vi "M07 Energy Storage.vi"(11 "NXT/EV3":T1) -> (3 "EV3 out":T1)   [LabVIEW 2016]
uses:
  <vilib>/NXT/Subs/LVHSConnector.ctl
  <vilib>/NXT/LegoClasses/BrickReference/BrickReference.lvclass
  <vilib>/NXT/Dual Mode Library/Waits/Wait_Num.vi
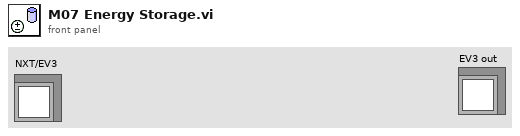
[diagram p1: front panel]
types:
  T1 = typedef "LVHSConnector.ctl" = refnum<class "BrickReference.lvclass">
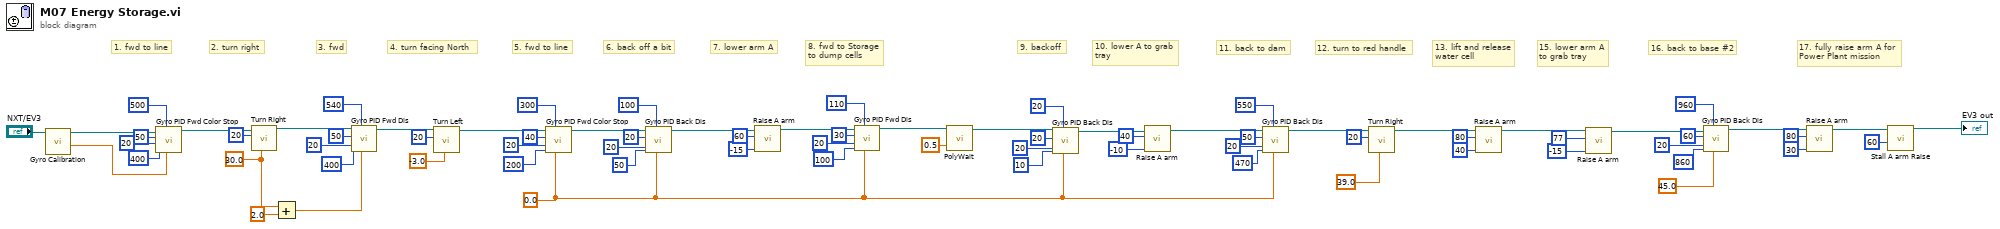
[diagram p0: block diagram]
diagram:
  w2 = sgl 0.0 ("Target angle")
  w35 = sgl 30.0 ("Turning angle")
  # "17. fully raise arm A for\nPower Plant mission"
  # "16. back to base #2"
  # "15. lower arm A\nto grab tray"
  # "13. lift and release\nwater cell"
  # "12. turn to red handle"
  # "11. back to dam"
  # "10. lower A to grab\ntray"
  # "9. backoff"
  # "8. fwd to Storage\nto dump cells"
  # "7. lower arm A"
  # "6. back off a bit"
  # "5. fwd to line"
  # "4. turn facing North"
  # "3. fwd"
  # "2. turn right"
  # "1. fwd to line"
  n1 = call "Gyro Calibration.vi"("NXT/EV3"="NXT/EV3") -> ("Degrees"=w71:sgl, "NXT/EV3"=w28:T1)  [unwired: 6 in, 1 out]
  n2 = call "Gyro PID Fwd Color Stop.vi"("Target angle"=w71, "Threshold to Color"=500, "Threshold to slow"=400, "Min. speed"=20, "Max. speed"=50, "EV3 in"=w28) -> ("EV3 out"=w70:T1)  [unwired: 5 in]
  n3 = call "Turn Right.vi"("Turning angle"=w35, "Motor B (right)"=i8 20, "EV3 in"=w70) -> ("EV3 out"=w68:T1)  [unwired: 8 in]
  n4 = Add(x=w35, y=sgl 2.0) -> (x+y=w33:sgl)
  n5 = call "Gyro PID Fwd Dis.vi"("Target angle"=w33, "Threshold to stop"=540, "Threshold to slow"=400, "Min. speed"=20, "Max. speed"=50, "EV3 in"=w68) -> ("EV3 out"=w63:T1)  [unwired: 5 in]
  n6 = call "Turn Left.vi"("Turning angle"=sgl -3.0, "Motor B (right)"=i8 20, "EV3 in"=w63) -> ("EV3 out"=w60:T1)  [unwired: 8 in]
  n7 = call "Gyro PID Fwd Color Stop.vi"("Target angle"=w2, "Threshold to Color"=300, "Threshold to slow"=200, "Min. speed"=20, "Max. speed"=40, "EV3 in"=w60) -> ("EV3 out"=w55:T1)  [unwired: 5 in]
  n8 = call "Gyro PID Back Dis.vi"("Target angle"=w2, "Threshold to stop"=100, "Threshold to slow"=50, "Min. speed"=20, "Max. speed"=20, "EV3 in"=w55) -> ("EV3 out"=w50:T1)  [unwired: 5 in]
  n9 = call "Raise A arm.vi"("Power"=i8 -15, "Rotation"=60, "EV3 in"=w50) -> ("EV3 out"=w47:T1)  [unwired: 8 in]
  n10 = call "Gyro PID Fwd Dis.vi"("Target angle"=w2, "Threshold to stop"=110, "Threshold to slow"=100, "Min. speed"=20, "Max. speed"=30, "EV3 in"=w47) -> ("EV3 out"=w42:T1)  [unwired: 5 in]
  n11 = call-poly <vilib>:"PolyWait.vi"("Time (1 sec)"=sgl 0.5, "NXT/EV3"=w42) -> ("NXT/EV3"=w40:T1)  [unwired: 2 in]
  n12 = call "Gyro PID Back Dis.vi"("Target angle"=w2, "Threshold to stop"=20, "Threshold to slow"=10, "Min. speed"=20, "Max. speed"=20, "EV3 in"=w40) -> ("EV3 out"=w31:T1)  [unwired: 5 in]
  n13 = call "Raise A arm.vi"("Power"=i8 -10, "Rotation"=40, "EV3 in"=w31) -> ("EV3 out"=w3:T1)  [unwired: 8 in]
  n14 = call "Gyro PID Back Dis.vi"("Target angle"=w2, "Threshold to stop"=550, "Threshold to slow"=470, "Min. speed"=20, "Max. speed"=50, "EV3 in"=w3) -> ("EV3 out"=w19:T1)  [unwired: 5 in]
  n15 = call "Turn Right.vi"("Turning angle"=sgl 39.0, "Motor B (right)"=i8 20, "EV3 in"=w19) -> ("EV3 out"=w9:T1)  [unwired: 8 in]
  n16 = call "Raise A arm.vi"("Power"=i8 40, "Rotation"=80, "EV3 in"=w9) -> ("EV3 out"=w17:T1)  [unwired: 8 in]
  n17 = call "Raise A arm.vi"("Power"=i8 -15, "Rotation"=77, "EV3 in"=w17) -> ("EV3 out"=w11:T1)  [unwired: 8 in]
  n18 = call "Gyro PID Back Dis.vi"("Target angle"=sgl 45.0, "Threshold to stop"=960, "Threshold to slow"=860, "Min. speed"=20, "Max. speed"=60, "EV3 in"=w11) -> ("EV3 out"=w6:T1)  [unwired: 5 in]
  n19 = call "Raise A arm.vi"("Power"=i8 30, "Rotation"=80, "EV3 in"=w6) -> ("EV3 out"=w5:T1)  [unwired: 8 in]
  n20 = call "Stall A arm Raise.vi"("Power"=i8 60, "NXT/EV3"=w5) -> ("NXT/EV3"=→"EV3 out":T1)  [unwired: 9 in]
